vi "init_Data.vi"(1 "Input":u8[](array[numeric]), 2 "Zerar CRC":bool) -> (0 "Output":u8[](array[numeric]))   [LabVIEW 2022 SP3]
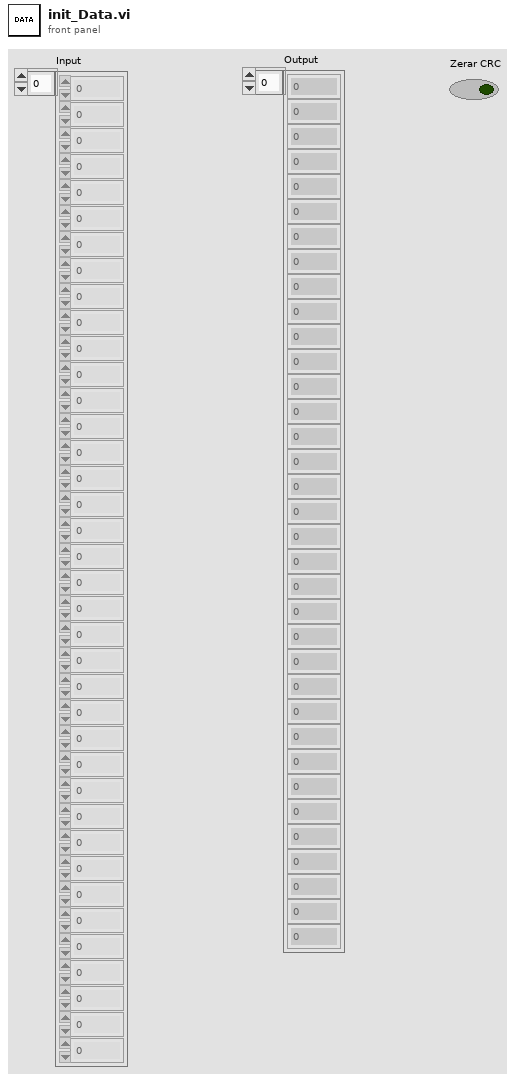
[diagram p1: front panel]
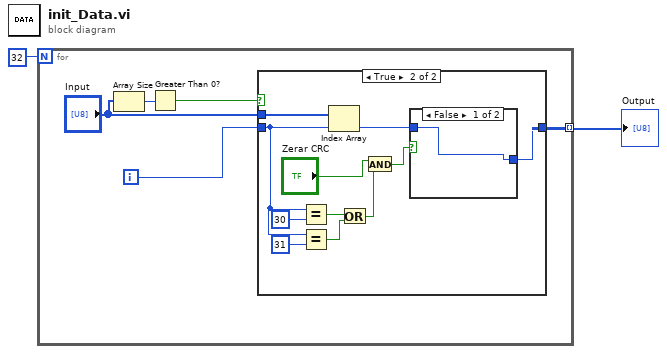
[diagram p0: block diagram]
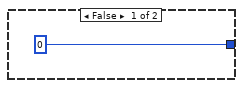
[diagram p2: hidden frame]
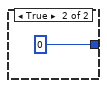
[diagram p3: hidden frame]
diagram:
  n1 = for {
    N: 32 -> [_]
    tunnel: [w6] -> w1 mode=indexing
    i -> [w7]
    n2 = Array Size(array="Input") -> (size(s)=w3:i32)
    n3 = Greater Than 0?(x=w3) -> (x > 0?=w4:bool)
    n4 = case shown="True" w4 {
      tunnel: w7 -> [_ w13]
      tunnel: [u8 0 ("Numeric") w10] -> w6
      tunnel: "Input" -> [_ w19]
      frame False {
      }
      frame True {
        n5 = Equal?(x=w13, y=30) -> (x = y?=w15:bool)
        n6 = Equal?(x=w13, y=31) -> (x = y?=w14:bool)
        n7 = Index Array(array=w19, index=w13) -> (element=w9:u8)
        n8 = Or(x=w15, y=w14) -> (x .or. y?=w16:bool)
        n9 = And(x="Zerar CRC", y=w16) -> (x .and. y?=w18:bool)
        n10 = case shown="False" w18 {
          tunnel: [w20 u8 0] -> w10
          tunnel: w9 -> [w20 _]
          frame False {
          }
          frame True {
          }
        }
      }
    }
  }
  "Output" <- w1
